vi "_API_TESTER.vi"() -> ()   [LabVIEW 2019, in "PredictiveMaintenance.lvlib"]
doc: "PMM API_TESTER:\nTo test API functions from Predictive Maintenance Module"
uses:
  PredictiveMaintenance.lvlib
  PredictiveMaintenance.lvclass
  C:/Program Files (x86)/National Instruments/LabVIEW 2019/vi.lib/ActorFramework/Actor/Actor.lvclass
  ConfigClass/_ConfigClass_INI/_ConfigClass_INI.lvclass
  PredictiveMaintenance.lvclass/PredictiveMaintenance.ctl
  <vilib>/ActorFramework/Message Enqueuer/Message Enqueuer.lvclass/Message Enqueuer.ctl
  PredictiveMaintenance Messages/SetEvent Msg/SetEvent Msg.lvclass/SetEvent Msg.ctl
  PredictiveMaintenance Messages/StartTrigger Msg/StartTrigger Msg.lvclass/StartTrigger Msg.ctl
  PredictiveMaintenance Messages/StopTrigger Msg/StopTrigger Msg.lvclass/StopTrigger Msg.ctl
  <vilib>/ActorFramework/Message Enqueuer/Enqueue.vi
  <vilib>/ActorFramework/Stop Msg/Stop Msg.lvclass
  C:/Program Files (x86)/National Instruments/LabVIEW 2019/vi.lib/ActorFramework/Message/Message.lvclass
  PredictiveMaintenance Messages/SetEvent Msg/SetEvent Msg.lvclass
  PredictiveMaintenance Messages/StartTrigger Msg/StartTrigger Msg.lvclass
  PredictiveMaintenance Messages/StopTrigger Msg/StopTrigger Msg.lvclass
  <vilib>/ActorFramework/Message Priority Queue/Priority Enqueue.vi
  <vilib>/ActorFramework/Actor/Actor.lvclass
  ConfigClass/ConfigClass/ConfigClass.lvclass
panel:
  out "error out":errorcluster
  in  "stop_trigger":bool
  in  "start_trigger":bool
  in  "Trigger":string
  in  "set_event":bool
  in  "Event":string
  in  "stop":bool
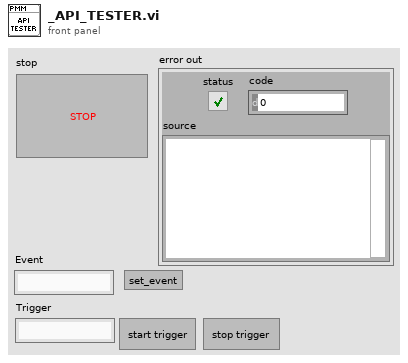
[diagram p1: front panel]
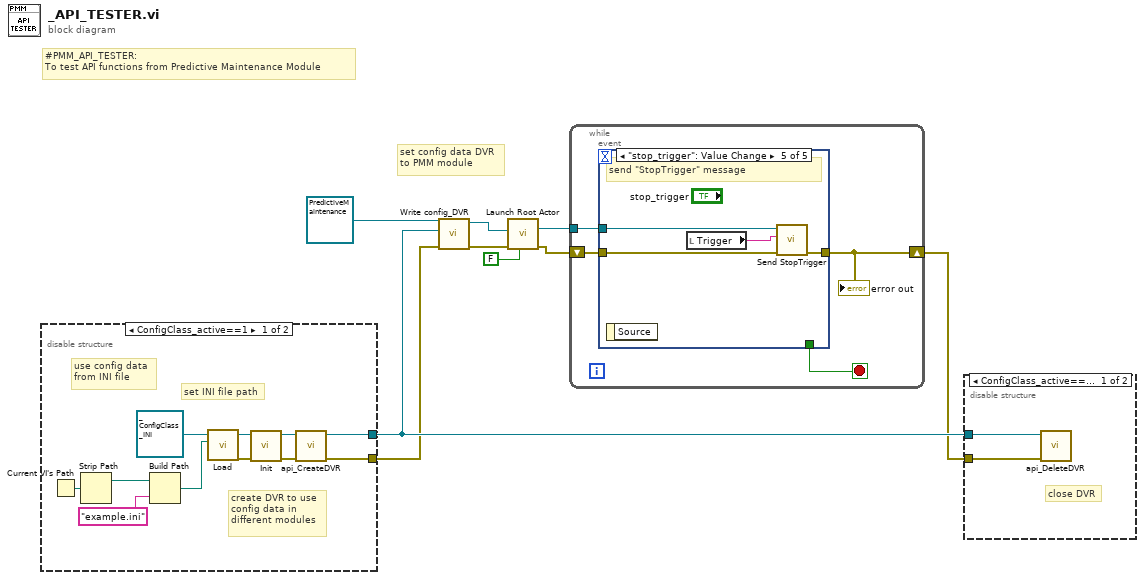
[diagram p0: block diagram]
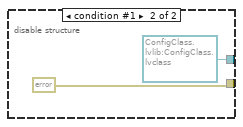
[diagram p3: hidden frame]
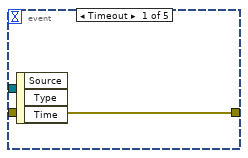
[diagram p4: hidden frame]
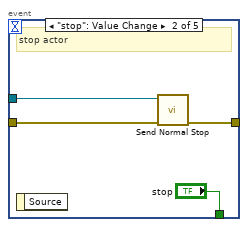
[diagram p5: hidden frame]
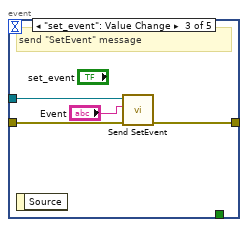
[diagram p6: hidden frame]
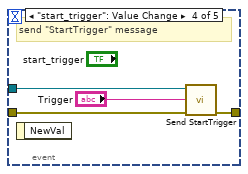
[diagram p7: hidden frame]
diagram:
  # "#PMM_API_TESTER:\nTo test API functions from Predictive Maintenance Module"
  # "set config data DVR\nto PMM module"
  n1 = disable-structure shown="ConfigClass_active==1" {
    disable-tunnel: [w20 refnum<data-value> refnum ("data value reference")] -> w6
    disable-tunnel: [w19 errorcluster {"status"=FALSE, "code"=0, "source"=""} ("error out")] -> w5
    frame condition #0 (active) {
      # "use config data\nfrom INI file"
      # "set INI file path"
      # "create DVR to use\nconfig data in\ndifferent modules"
      n2 = Current VI's Path() -> (path=w13:path)
      n3 = Strip Path(path=w13) -> (stripped path=w12:path)  [unwired: 1 out]
      n4 = Build Path(base path=w12, name or relative path="example.ini") -> (appended path=w10:path)
      n5 = call-dynamic "Load.vi"("Data_IN"=w10, "_ConfigClass_INI_IN"=refnum<class "_ConfigClass_INI.lvclass"> refnum ("_ConfigClass_INI.lvlib:_ConfigClass_INI.lvclass")) -> ("error out"=w15:errorcluster, "_ConfigClass_INI_OUT"=w18:refnum<class "_ConfigClass_INI.lvclass">)  [unwired: 8 in]
      n6 = call-dynamic "Init.vi"("error in (no error)"=w15, "Config.lvlib:_ConfigClass_ApplSett_IN"=w18) -> ("error out"=w14:errorcluster, "Config.lvlib:_ConfigClass_ApplSett_OUT"=w16:refnum<class "_ConfigClass_INI.lvclass">)  [unwired: 8 in]
      n7 = call-dynamic "api_CreateDVR.vi"("error in (no error)"=w14, "ConfigClass.lvlib:ConfigClass.lvclass"=w16) -> ("error out"=w19:errorcluster, "data value reference"=w20:refnum<data-value>)  [unwired: 8 in]
    }
    frame condition #1 {
    }
  }
  n8 = call "Write config_DVR.vi"("error in (no error)"=w5, "config_DVR"=w6, "PredictiveMaintenance.lvlib:PredictiveMaintenance.lvclass"=refnum<class "PredictiveMaintenance.lvclass"> refnum) -> ("error out"=w4:errorcluster, "PredictiveMaintenance.lvlib:PredictiveMaintenance.lvclass 2"=w7:refnum<class "PredictiveMaintenance.lvclass">)  [unwired: 7 in]
  n9 = call <vilib>:"Launch Root Actor.vi"("Open Actor Core front panel? (F)"=FALSE, "error in (no error)"=w4, "Actor"=w7) -> ("error out"=w2:errorcluster, "Actor's Enqueuer"=w9:refnum<class "Message Enqueuer.lvclass">)  [unwired: 7 in]
  n10 = while {
    tunnel: w9 -> [w25]
    shift-right: [w24] -> w3
    shift-left: w2 -> [w23]
    stop <- w26 stop-if-true
    n11 = event shown="[4] \"stop_trigger\": Value Change" {
      selector: _ -> [_ _ _ _ _]
      dyn-events: _ -> [_ _ _ _ _]
      timeout: _ -> [_ _ _ _ _]
      tunnel: [_ "stop" _ _ _] -> w26
      tunnel: w25 -> [_ w30 w35 w39 w43]
      tunnel: [w27 w28 w33 w38 w42] -> w24
      tunnel: w23 -> [w27 w29 w32 w37 w41]
      event Timeout {
        n12 = event-data() -> ()  [unwired: 1 in, 3 out]
      }
      event "stop": Value Change {
        # "stop actor"
        n13 = event-data() -> ()  [unwired: 1 in, 1 out]
        n14 = call <vilib>:"Send Normal Stop.vi"("error in (no error)"=w29, "Message Enqueuer"=w30) -> ("error out"=w28:errorcluster)  [unwired: 9 in]
      }
      event "set_event": Value Change {
        # "send \"SetEvent\" message"
        n15 = event-data() -> ()  [unwired: 1 in, 1 out]
        n16 = call "Send SetEvent.vi"("error in (no error)"=w32, "event"="Event", "Message Enqueuer"=w35) -> ("error out"=w33:errorcluster)  [unwired: 7 in, 1 out]
      }
      event "start_trigger": Value Change {
        # "send \"StartTrigger\" message"
        n17 = event-data() -> ()  [unwired: 1 in, 1 out]
        n18 = call "Send StartTrigger.vi"("error in (no error)"=w37, "trigger"="Trigger", "Message Enqueuer"=w39) -> ("error out"=w38:errorcluster)  [unwired: 7 in, 1 out]
      }
      event "stop_trigger": Value Change {
        # "send \"StopTrigger\" message"
        n19 = event-data() -> ()  [unwired: 1 in, 1 out]
        n20 = local read "Trigger"() -> (w40:string)
        n21 = call "Send StopTrigger.vi"("error in (no error)"=w41, "trigger"=w40, "Message Enqueuer"=w43) -> ("error out"=w42:errorcluster)  [unwired: 7 in, 1 out]
      }
    }
    "error out" <- w24
  }
  n22 = disable-structure shown="ConfigClass_active==1" {
    disable-tunnel: w6 -> [w45 _]
    disable-tunnel: w3 -> [w44 _]
    frame condition #0 (active) {
      # "close DVR"
      n23 = call "api_DeleteDVR.vi"("error in (no error)"=w44, "data value reference"=w45) -> ()  [unwired: 9 in, 1 out]
    }
    frame condition #1 {
    }
  }
